vi "majorcheck.vi"(11 "Array in":bool[](array[boolean])) -> (3 "Array out":bool[](array[boolean]))   [LabVIEW 2019]
uses:
  <vilib>/Utility/file.llb/Read Delimited Spreadsheet (string).vi
panel:
  out "all rows":string[][](array[string])
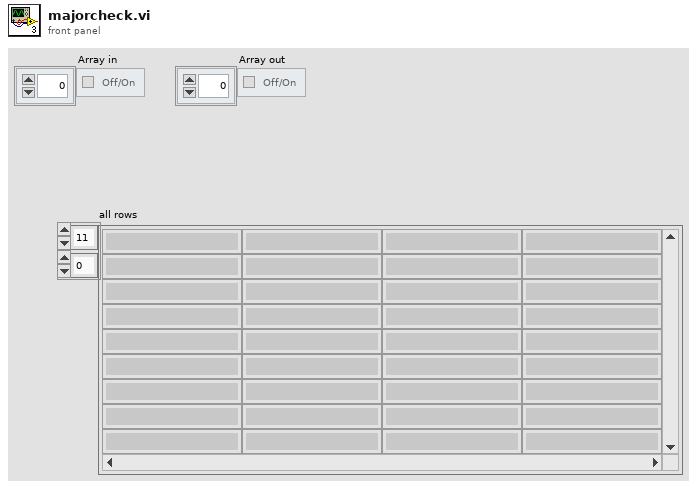
[diagram p1: front panel]
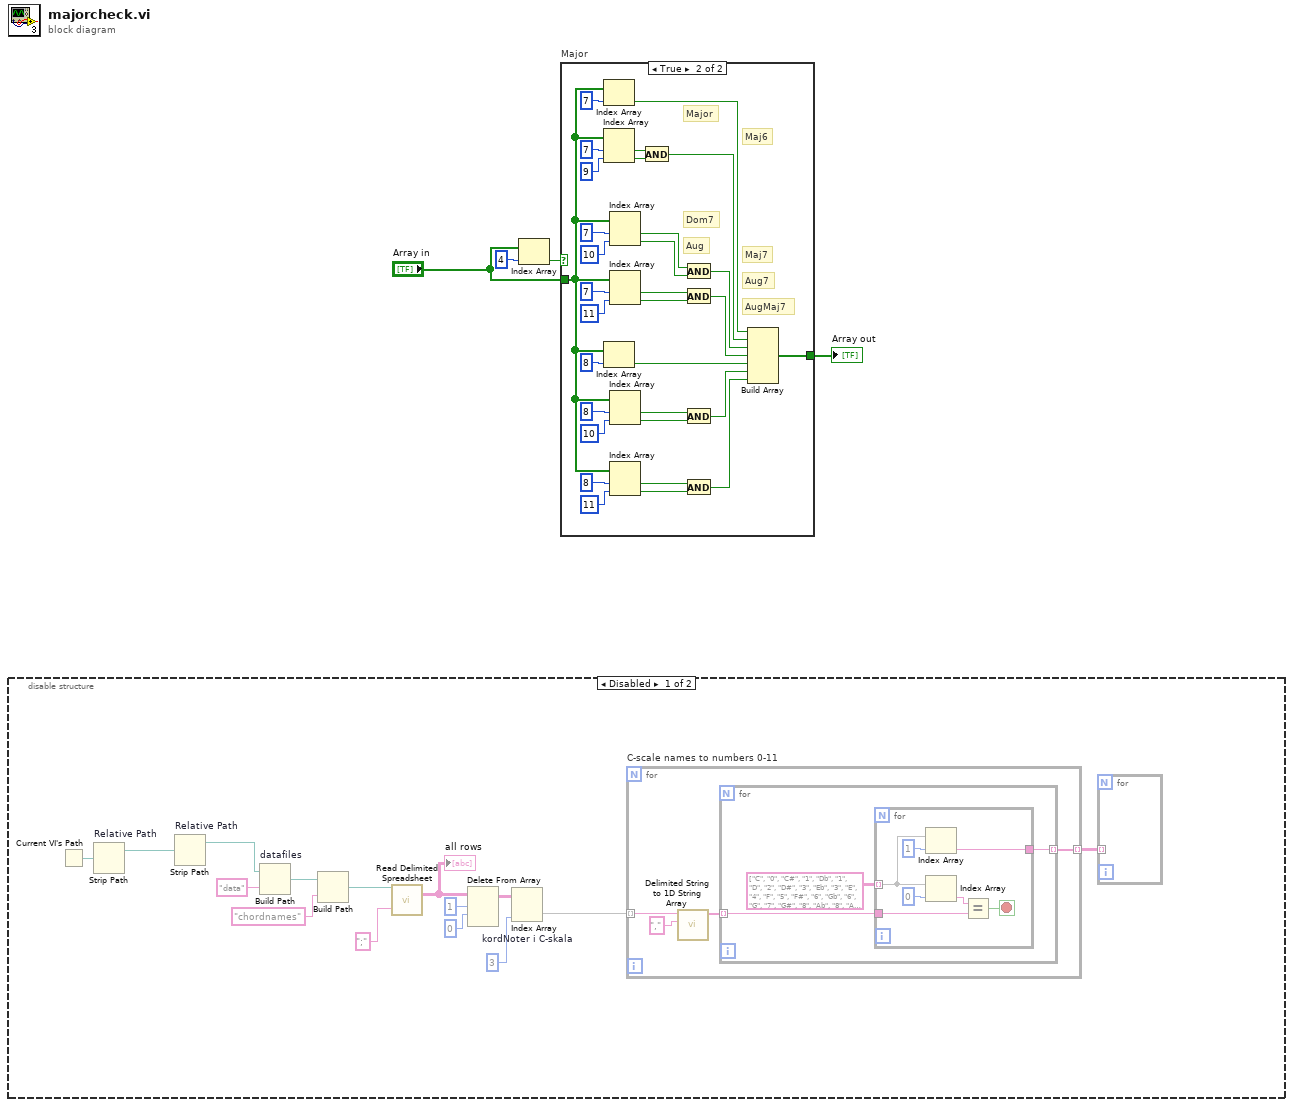
[diagram p0: block diagram]
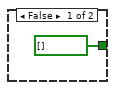
[diagram p3: hidden frame]
diagram:
  n1 = disable-structure shown="Disabled" {
    frame Disabled {
      n2 = Current VI's Path() -> (path=w18:path)
      n3 = Strip Path "Relative Path"(path=w18) -> (stripped path=w14:path)  [unwired: 1 out]
      n4 = Strip Path "Relative Path"(path=w14) -> (stripped path=w13:path)  [unwired: 1 out]
      n5 = Build Path "datafiles"(base path=w13, name or relative path="data") -> (appended path=w15:path)
      n6 = Build Path(base path=w15, name or relative path="chordnames") -> (appended path=w12:path)
      n7 = call-poly <vilib>:"Read Delimited Spreadsheet.vi"("file path (dialog if empty)"=w12, "delimiter (\\t)"=";" ("delimiter (\\t)")) -> ("all rows"=w9:string[][])  [unwired: 8 in, 5 out]
      "all rows" <- w9
      n8 = Delete From Array(array=w9, length=1, index (row)=0) -> (array with subset deleted=w8:string[][])  [unwired: 1 in, 1 out]
      n9 = Index Array "kordNoter i C-skala"(array=w8, index (col)=3 ("index (row)")) -> (element=w6:string[])  [unwired: 1 in]
      n10 = for "C-scale names to numbers 0-11" {
        tunnel: w6 -> [w23] mode=indexing
        tunnel: [w20] -> w5 mode=indexing
        n11 = call <vilib>:"Delimited String to 1D String Array.vi"("delimiter"=",", "delimited string"=w23) -> ("string array"=w21:string[])  [unwired: 9 in]
        n12 = for {
          tunnel: w21 -> [w25] mode=indexing
          tunnel: [w24] -> w20 mode=indexing
          n13 = for {
            tunnel: string[][] [["C", "0"], ["C#", "1"], ["Db", "1"], ["D", "2"], ["D#", "3"], ["Eb", "3"], ["E", "4"], ["F", "5"], ["F#", "6"], ["Gb", "6"], ["G", "7"], ["G#", "8"], ["Ab", "8"], ["A", "9"], ["A#", "10"], ["Bb", "10"], ["B", "11"]] -> [w31] mode=indexing
            tunnel: w25 -> [w29]
            tunnel: [w28] -> w24
            stop <- w27 stop-if-true
            n14 = Index Array(array=w31, index=1) -> (element=w28:string)
            n15 = Index Array(array=w31, index=0) -> (element=w32:string)
            n16 = Equal?(x=w32, y=w29) -> (x = y?=w27:bool)
          }
        }
      }
      n17 = for {
        tunnel: w5 -> [_] mode=indexing
      }
    }
    frame Enabled {
    }
  }
  n18 = Index Array(array="Array in", index=4) -> (element=w3:bool)
  n19 = case "Major" shown="True" w3 {
    tunnel: "Array in" -> [_ w39]
    tunnel: [bool[] [] w41] -> w2
    frame False {
    }
    frame True {
      # "AugMaj7"
      # "Aug7"
      # "Aug"
      # "Maj7"
      # "Maj6"
      # "Dom7"
      # "Major"
      n20 = Index Array(array=w39, index=7) -> (element=w47:bool)
      n21 = Index Array(array=w39, index #1=7 ("index"), index #2=9 ("index")) -> (element #1=w57:bool, element #2=w58:bool)
      n22 = Index Array(array=w39, index=8) -> (element=w43:bool)
      n23 = Index Array(array=w39, index #1=7 ("index"), index #2=10 ("index")) -> (element #1=w62:bool, element #2=w61:bool)
      n24 = Index Array(array=w39, index #1=7 ("index"), index #2=11 ("index")) -> (element #1=w55:bool, element #2=w49:bool)
      n25 = Index Array(array=w39, index #1=8 ("index"), index #2=10 ("index")) -> (element #1=w48:bool, element #2=w50:bool)
      n26 = Index Array(array=w39, index #1=8 ("index"), index #2=11 ("index")) -> (element #1=w36:bool, element #2=w37:bool)
      n27 = And(x=w57, y=w58) -> (x .and. y?=w46:bool)
      n28 = And(x=w62, y=w61) -> (x .and. y?=w45:bool)
      n29 = And(x=w55, y=w49) -> (x .and. y?=w44:bool)
      n30 = And(x=w48, y=w50) -> (x .and. y?=w42:bool)
      n31 = And(x=w36, y=w37) -> (x .and. y?=w35:bool)
      n32 = Build Array(w47, w46, w45, w44, w43, w42, w35) -> (w41:bool[])
    }
  }
  "Array out" <- w2
